vi "spec_GetData.vi"(8 "error in (no error)":errorcluster, 10 "Detector":string, 11 "Qtegra in":refnum<class "Qtegra.lvclass">) -> (0 "error out":errorcluster, 1 "failed?":bool, 2 "value":dbl, 3 "Qtegra out":refnum<class "Qtegra.lvclass">)   [LabVIEW 2017, in "Qtegra.lvclass"]
doc: "reads the current value of the detector of the selected spectrometer"
uses:
  Qtegra.lvclass
  \\Mac\Home/my data/University/Lamont/Software/LabView/MSControlSuite_Code/MSControl/Classes/Instrument/instrument.lvclass
  global variables.vi
  instrument.lvclass
  StatusLog/StatusLog.lvclass
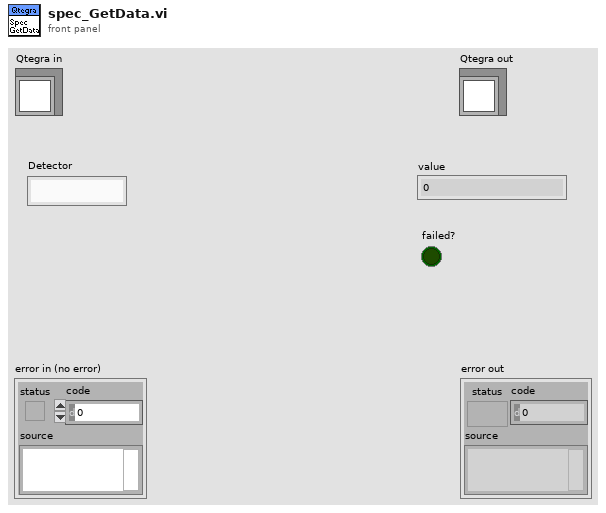
[diagram p1: front panel]
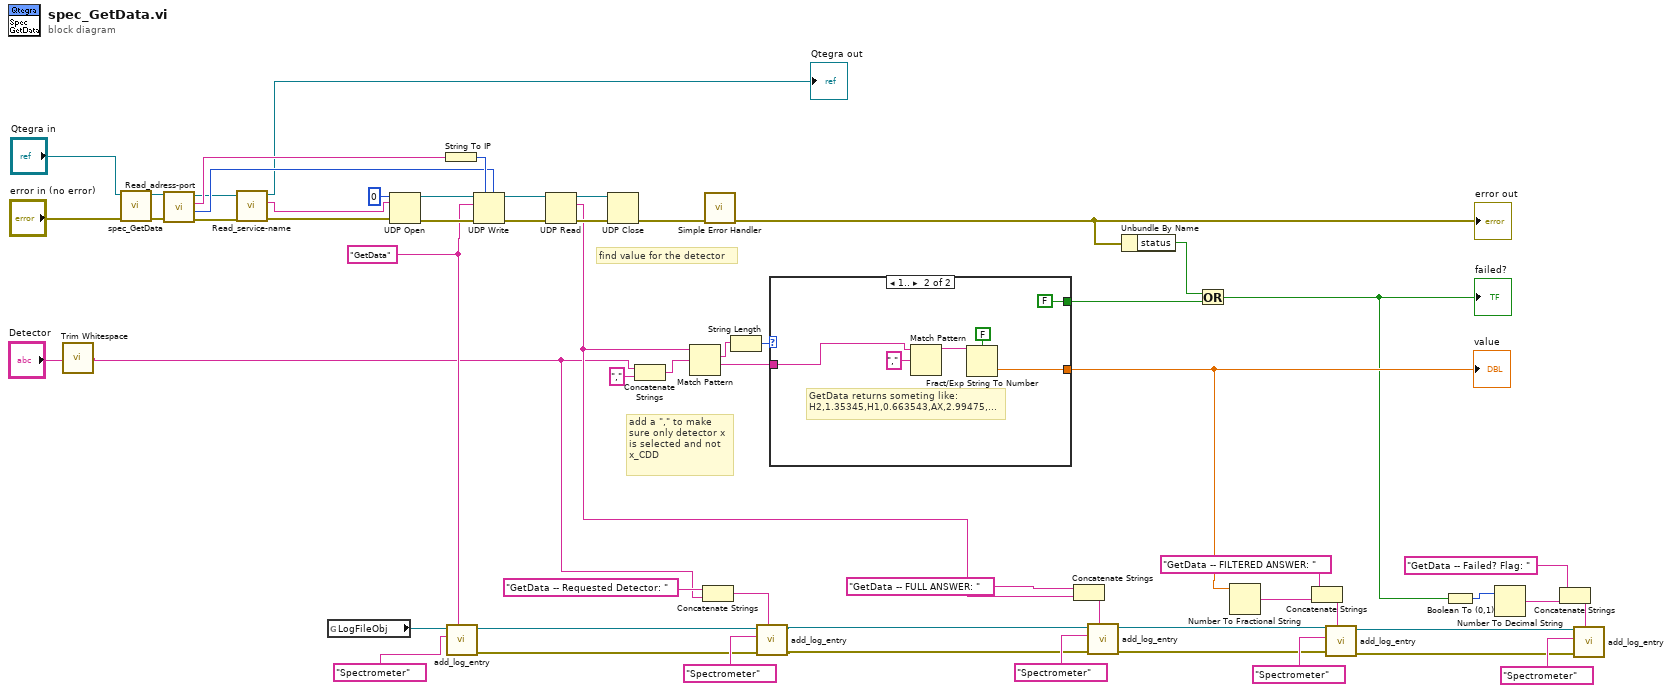
[diagram p0: block diagram]
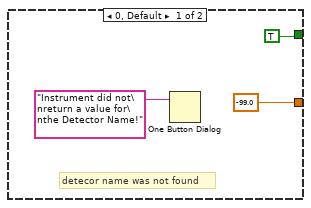
[diagram p2: hidden frame]
diagram:
  w29 = "GetData" ("format string")
  # "add a \",\" to make\nsure only detector x\nis selected and not\nx_CDD"
  # "find value for the detector"
  n1 = call <vilib>:"Trim Whitespace.vi"("string"="Detector") -> ("trimmed string"=w13:string)  [unwired: 1 in]
  n2 = call-parent "spec_GetData.vi"("error in (no error)"="error in (no error)", "instrument in"="Qtegra in") -> ("error out"=w41:errorcluster, "instrument out"=w42:refnum<class "Qtegra.lvclass">)  [unwired: 6 in, 2 out]
  n3 = call "Read_adress-port.vi"("error in (no error)"=w41, "instrument in"=w42) -> ("error out"=w49:errorcluster, "port number"=w50:i32, "adress"=w57:string, "instrument out"=w48:refnum<class "Qtegra.lvclass">)  [unwired: 6 in]
  n4 = call-dynamic "Read_service-name.vi"("error in (no error)"=w49, "instrument in"=w48) -> ("error out"=w47:errorcluster, "service name"=w46:string, "instrument out"=→"Qtegra out":refnum<class "Qtegra.lvclass">)  [unwired: 7 in]
  n5 = global read "global variables.vi" "LogFileObj"() -> (w34:refnum<class "StatusLog.lvclass">)
  n6 = UDP Open(8:w47, 10:w46, 11:u16 0 ("port")) -> (port=w53:refnum<k16>, 0:w54:errorcluster)  [unwired: 2 in, 1 out]
  n7 = String To IP(1:w57) -> (0:w56:u32)
  n8 = call-dynamic "add_log_entry.vi"("new entry"=w29, "log identifiers"="Spectrometer", "StatusLog in"=w34) -> ("error out"=w30:errorcluster, "StatusLog out"=w33:refnum<class "StatusLog.lvclass">)  [unwired: 5 in]
  n9 = UDP Write(address=w56, port or service name=w50, connection ID=w53, data in=w29, 8:w54) -> (error out=w51:errorcluster, 3:w52:refnum<k16>)  [unwired: 1 in]
  n10 = UDP Read(connection ID=w52, 8:w51) -> (data out=w23:string, error out=w45:errorcluster, 3:w43:refnum<k16>)  [unwired: 2 in, 2 out]
  n11 = UDP Close(connection ID=w43, 8:w45) -> (error out=w44:errorcluster)  [unwired: 1 out]
  n12 = Concatenate Strings(w13, "," ("string")) -> (w14:string)
  n13 = Match Pattern(string=w23, regular expression=w14) -> (match substring=w38:string, after substring=w39:string)  [unwired: 1 in, 2 out]
  n14 = Concatenate Strings("GetData -- Requested Detector: ", w13) -> (w31:string)
  n15 = call <vilib>:"Simple Error Handler.vi"("error in (no error)"=w44) -> ("error out"=w11:errorcluster)  [unwired: 4 in, 4 out]
  "error out" <- w11
  n16 = String Length(string=w38) -> (length=w37:i32)
  n17 = call-dynamic "add_log_entry.vi"("new entry"=w31, "error in (no error)"=w30, "log identifiers"="Spectrometer", "StatusLog in"=w33) -> ("error out"=w25:errorcluster, "StatusLog out"=w26:refnum<class "StatusLog.lvclass">)  [unwired: 4 in]
  n18 = case shown="1.." w37 {
    tunnel: w39 -> [_ w64]
    tunnel: [-99.0 w67] -> w16
    tunnel: [TRUE FALSE] -> w9
    frame 0, Default {
      # "detecor name was not found"
      n19 = One Button Dialog(message="Instrument did not\nreturn a value for\nthe Detector Name!") -> ()  [unwired: 1 in, 1 out]
    }
    frame 1.. {
      # "GetData returns someting like:\nH2,1.35345,H1,0.663543,AX,2.99475,..."
      n20 = Match Pattern(string=w64, regular expression=",") -> (before substring=w68:string)  [unwired: 1 in, 3 out]
      n21 = Fract/Exp String To Number(use system decimal point (T)=FALSE, string=w68) -> (number=w67:dbl)  [unwired: 2 in, 1 out]
    }
  }
  "value" <- w16
  n22 = Concatenate Strings("GetData -- FULL ANSWER: ", w23) -> (w28:string)
  n23 = call-dynamic "add_log_entry.vi"("new entry"=w28, "error in (no error)"=w25, "log identifiers"="Spectrometer", "StatusLog in"=w26) -> ("error out"=w19:errorcluster, "StatusLog out"=w20:refnum<class "StatusLog.lvclass">)  [unwired: 4 in]
  n24 = Unbundle By Name(w11) -> ("status"=w10:bool)
  n25 = Or(x=w10, y=w9) -> (x .or. y?=w1:bool)
  "failed?" <- w1
  n26 = Number To Fractional String(number=w16) -> (F-format string=w17:string)  [unwired: 3 in]
  n27 = Concatenate Strings("GetData -- FILTERED ANSWER: ", w17) -> (w21:string)
  n28 = call-dynamic "add_log_entry.vi"("new entry"=w21, "error in (no error)"=w19, "log identifiers"="Spectrometer", "StatusLog in"=w20) -> ("error out"=w5:errorcluster, "StatusLog out"=w6:refnum<class "StatusLog.lvclass">)  [unwired: 4 in]
  n29 = Boolean To (0,1)(Boolean=w1) -> (0, 1=w3:i16)
  n30 = Number To Decimal String(number=w3) -> (decimal integer string=w2:string)  [unwired: 1 in]
  n31 = Concatenate Strings("GetData -- Failed? Flag: ", w2) -> (w8:string)
  n32 = call-dynamic "add_log_entry.vi"("new entry"=w8, "error in (no error)"=w5, "log identifiers"="Spectrometer", "StatusLog in"=w6) -> ()  [unwired: 4 in, 2 out]
